vi "Is Support Hard Trigger.vi"() -> (3 "function return":i32)   [LabVIEW 2021, in "vmmso.lvlib"]
doc: "DLL_API int WINAPI IsSupportHardTrigger();"
uses:
  vmmso.lvlib
  vmmso.dll
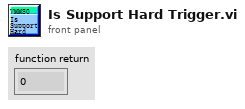
[diagram p1: front panel]
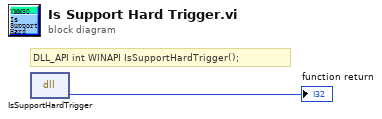
[diagram p0: block diagram]
diagram:
  # "DLL_API int WINAPI IsSupportHardTrigger();"
  n1 = dll-call lib="D:/labviewdemo/LabviewDemo 21/vmmso/vmmso.*" fn="IsSupportHardTrigger"() -> (→"function return":i32)  [unwired: 3 in, 2 out]
